vi "RT.vi"() -> ()   [LabVIEW 2013]
uses:
  ieeeC37_118.dll
  pmuConnectionData.dll
  <vilib>/rvi/interface/nirviOpenFPGA/nirviOpenFPGA.xnode
  <vilib>/rvi/interface/nirviReadWriteControl/nirviReadWriteControl.xnode
  <vilib>/rvi/interface/nirviCloseFPGA/nirviCloseFPGA.xnode
  <vilib>/FPGAPlugInAG/Dynamic/niLvFpga_Close_Dynamic.vi
  FPGA Bitfiles/AudurPhasorPodKh_FPGATarget_FPGA_S0BGwwaa7CI.lvbitx
  FPGA.vi
  <vilib>/FPGAPlugInAG/cRIO-9081/niLvFpga_Open_cRIO-9081.vi
  <vilib>/rvi/interface/common/dynamic/niFpgaDynamicAddResources.vi
  NiFpgaLv.dll
  <vilib>/Utility/error.llb/Error Cluster From Error Code.vi
  <vilib>/rvi/interface/Simulation/niFpgaSimulationCallBeginRW.vi
  <vilib>/rvi/errors/niLvFpgaAdjustHostInterfaceError.vi
panel:
  in  "Scaling":sgl
  in  "Alpha":sgl
  in  "Freq of Osc":sgl
  out "FPGA error":errorcluster
  out "Samples\nReceived":i32
  in  "Tab Control 4":enum32{"PMUs Data Stream"}(tab)
  out "Frequency":sgl[](array[numeric])
  out "ROCOF":sgl[](array[numeric])
  out "Phasors\n(Magnitude)":sgl[](array[numeric])
  out "Phasors\n(Angle-Degree)":sgl[](array[numeric])
  out "Data Time Stamp":T1
  out "Analogs\n(Value)":sgl[](array[numeric])
  out "Phasors\n(Channel Names)":string[](array[string])
  out "Phasors\n(Types)":string[](array[string])
  out "Phasors\n(PMU Names)":string[](array[string])
  out "Analogs\n(Channel Names)":string[](array[string])
  out "Analogs\n(Types)":string[](array[string])
  out "Analogs\n(PMU Names)":string[](array[string])
  out "Data Error Status":string[](array[string])
  out "PMU Sync Status":string[](array[string])
  out "Data Processed":string[](array[string])
  out "PMU Time Quality":string[](array[string])
  out "PMU Unlocked Time":string[](array[string])
  out "PMU Triggered":string[](array[string])
  out "Trigger Reason":string[](array[string])
  in  "Tab Control 3":enum32{"Connection Data"}(tab)
  in  "IP Address (PMU / PDC)":string="130.237.53.177"
  in  "ID CODE":i32=787
  in  "Port Number":i32=38068
  in  "Tab Control 2":enum32{"PMUs Configuration"}(tab)
  out "Number of\nAnalogs":u16[](array[numeric])
  out "Number of\nDigitals":u16[](array[numeric])
  out "Nominal\nFrequency":sgl[](array[numeric])
  out "Configuration\nCount":u16[](array[numeric])
  out "Number of\nPhasors":u16[](array[numeric])
  out "Station\nName":string[](array[string])
  out "ID Code":u16[](array[numeric])
  in  "Tab Control":enum32{"PDC Configuration"}(tab)
  out "Data Rate:":u16
  out "Number of PMUs:":u16
  out "Configuration Time Stamp":T2
  in  "Shut Down":bool
  out "error out":errorcluster
  # "FPGA Controlls"
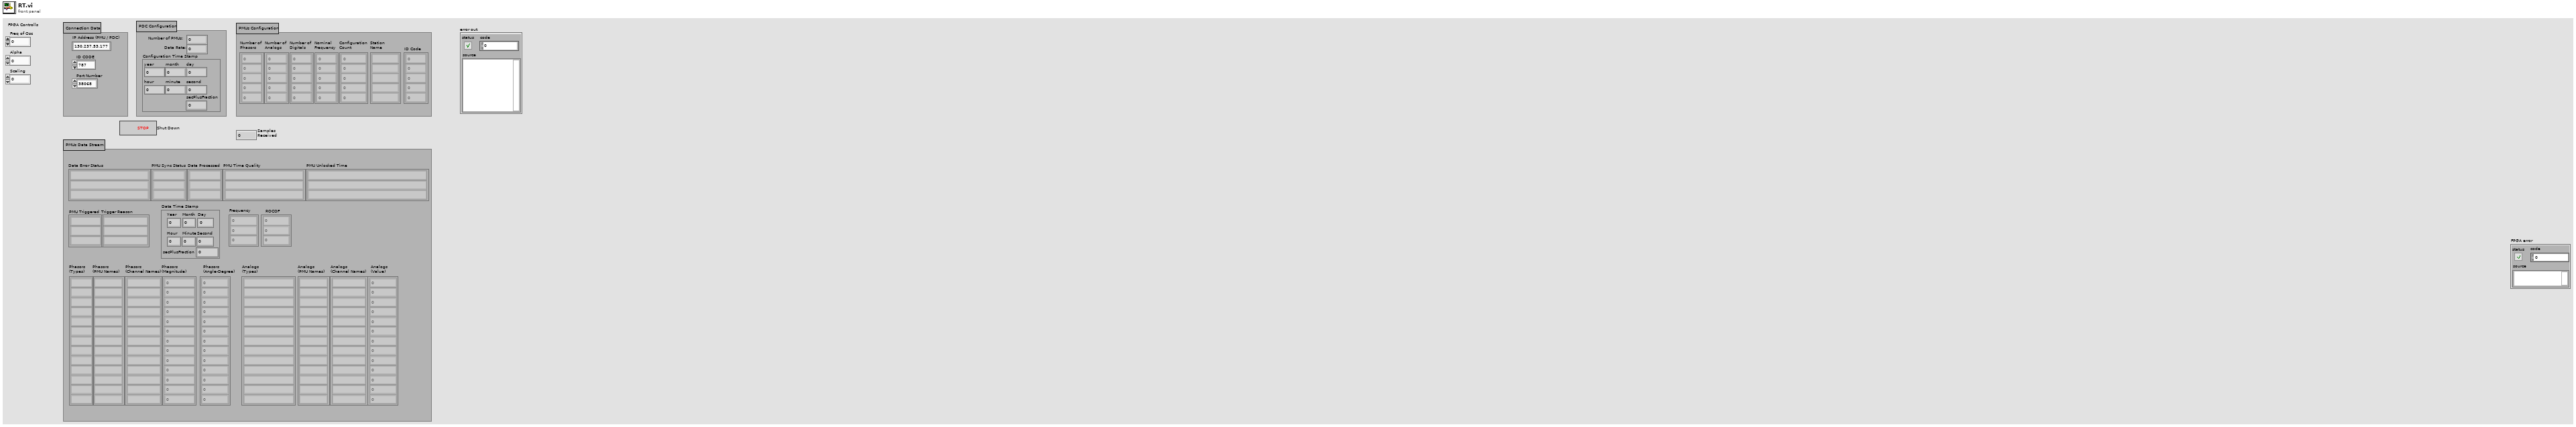
[diagram p1: front panel]
types:
  T1 = cluster{"Year":i32, "Month":i32, "Day":i32, "Hour":i32, "Minute":i32, "Second":i32, "secPlusFraction":sgl}
  T2 = cluster{"year":i32, "month":i32, "day":i32, "hour":i32, "minute":i32, "second":i32, "secPlusFraction":sgl}
  T3 = cluster{"dataError":u8, "dataModified":u8, "pmuIsNOTSync":u8, "pmuIsTriggered":u8, "pmuTimeQuality":u8, "triggerReason":u8, "unlockTime":u8}
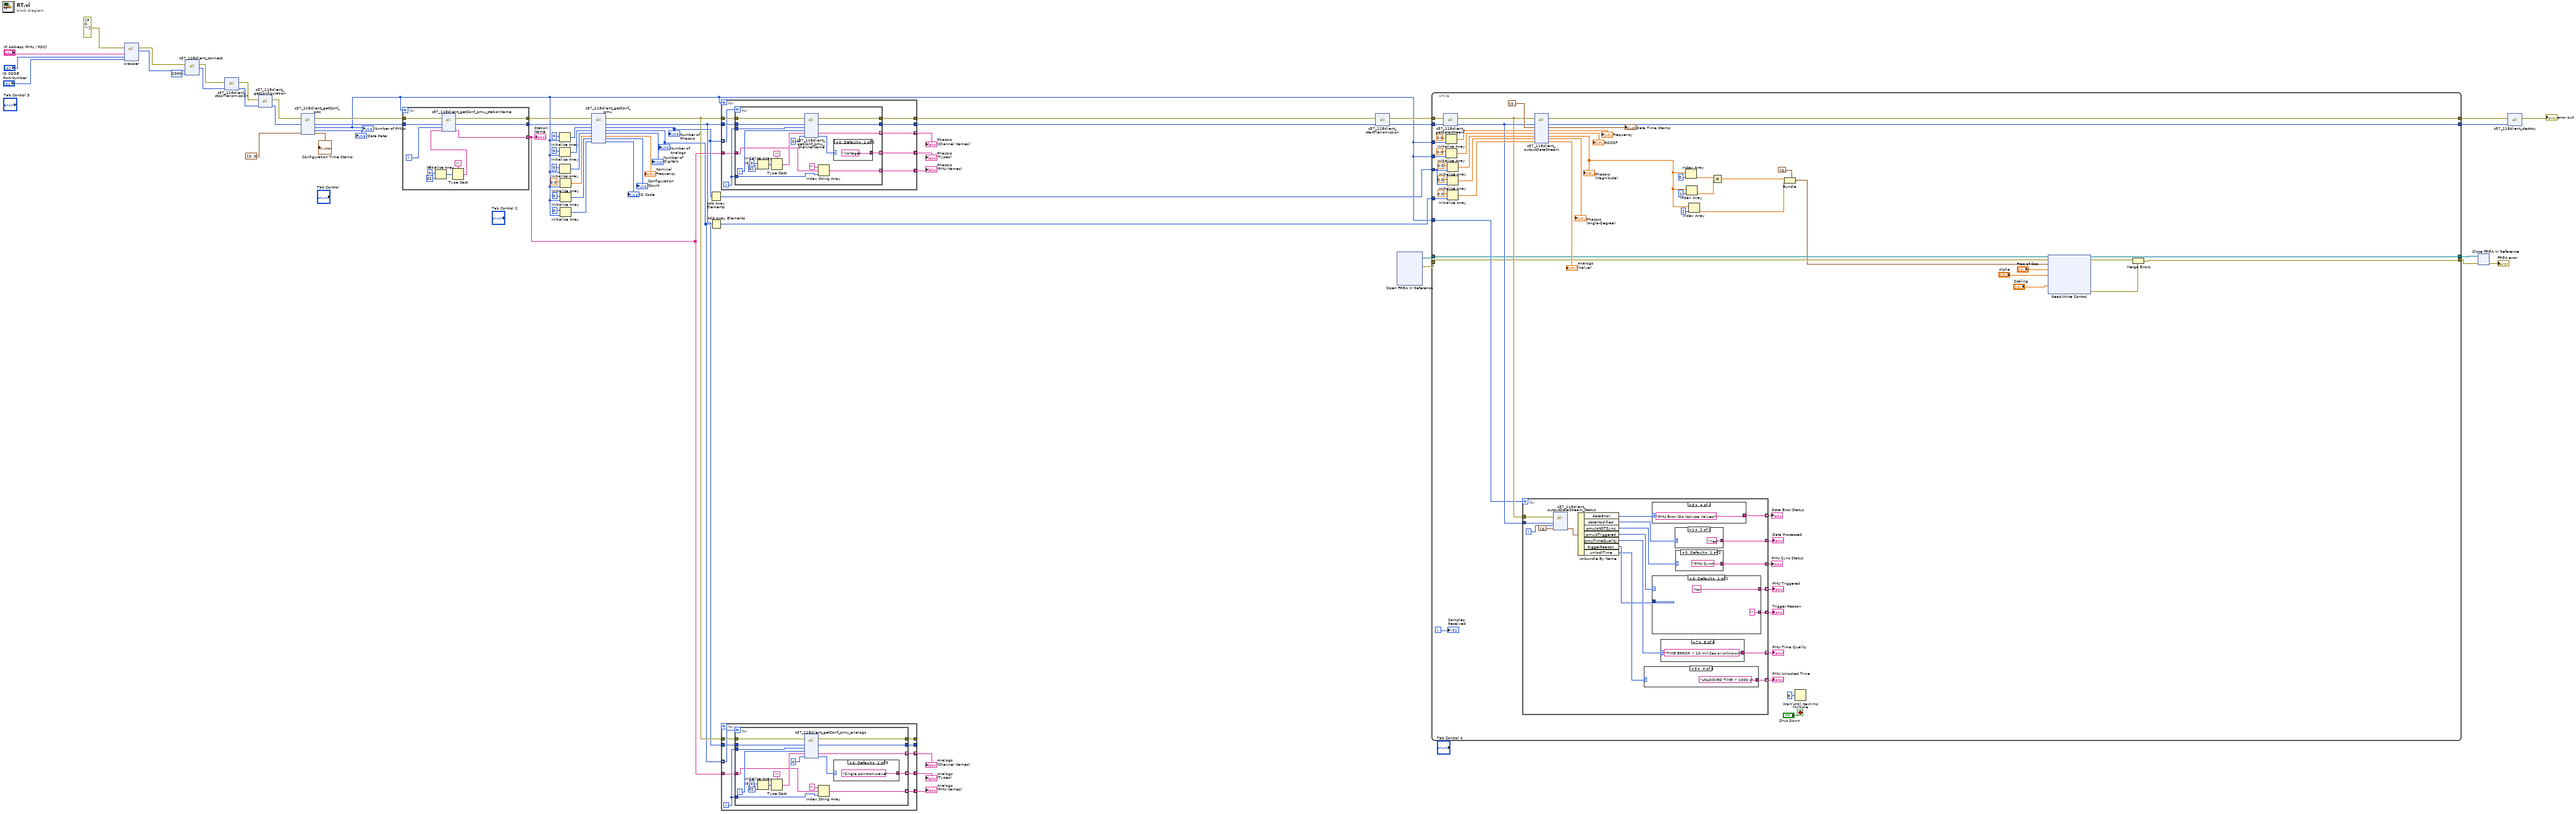
[diagram p0: block diagram]
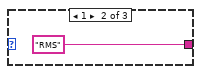
[diagram p2: hidden frame]
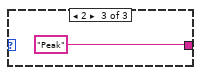
[diagram p3: hidden frame]
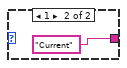
[diagram p4: hidden frame]
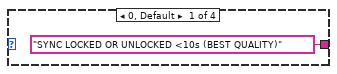
[diagram p5: hidden frame]
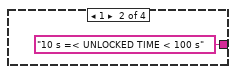
[diagram p6: hidden frame]
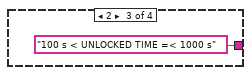
[diagram p7: hidden frame]
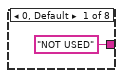
[diagram p8: hidden frame]
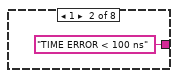
[diagram p9: hidden frame]
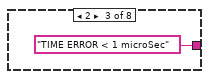
[diagram p10: hidden frame]
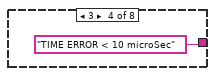
[diagram p11: hidden frame]
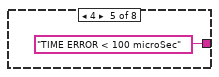
[diagram p12: hidden frame]
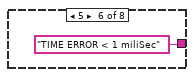
[diagram p13: hidden frame]
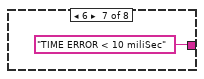
[diagram p14: hidden frame]
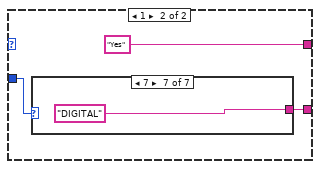
[diagram p15: hidden frame]
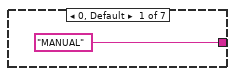
[diagram p16: hidden frame]
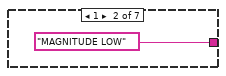
[diagram p17: hidden frame]
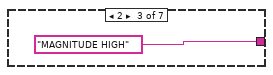
[diagram p18: hidden frame]
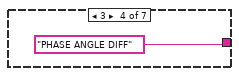
[diagram p19: hidden frame]
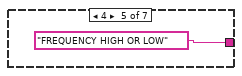
[diagram p20: hidden frame]
diagram:
  n1 = dll-call lib="pmuConnectionData.*" fn="wrapper"(error in=errorcluster {"status"=FALSE, "code"=0, "source"=""} ("error in (no error)"), "ipAddress_PmuServer"="IP Address (PMU / PDC)", "pmuPortNumber"="ID CODE", "pmuIdCode"="Port Number") -> (error out=w53:errorcluster, "PMUConnectionData"=w62:i64)  [unwired: 5 in, 1 out]
  n2 = dll-call lib="ieeeC37_118.*" fn="c37_118client_connect"(error in=w53, "parameters"=w62, "timeoutInMs"=u32 2000) -> (error out=w52:errorcluster, "c37_118Object"=w60:i64)  [unwired: 4 in, 1 out]
  n3 = dll-call lib="ieeeC37_118.dll" fn="c37_118client_stopTransmission"(error in=w52, "self"=w60) -> (error out=w51:errorcluster, "self"=w59:i64)  [unwired: 3 in, 1 out]
  n4 = dll-call lib="ieeeC37_118.dll" fn="c37_118client_getConfiguration"(error in=w51, "self"=w59) -> (error out=w50:errorcluster, "self"=w56:i64)  [unwired: 3 in, 1 out]
  n5 = dll-call lib="ieeeC37_118.dll" fn="c37_118client_getConf_pdc"(error in=w50, "self"=w56, "timestamp"=T2 {"year"=0, "month"=0, "day"=0, "hour"=0, "minute"=0, "second"=0, "secPlusFraction"=0.0}) -> (error out=w27:errorcluster, "self"=w25:i64, "num_pmu"=w6:u16, "data_rate"=→"Data Rate:":u16, "timestamp"=→"Configuration Time Stamp":T2)  [unwired: 5 in, 1 out]
  "Number of PMUs:" <- w6
  n6 = for {
    N: w6 -> [_]
    tunnel: w27 -> [w73]
    tunnel: [w72] -> w26
    tunnel: w25 -> [w71]
    tunnel: [w70] -> w24
    tunnel: [w69] -> w10 mode=indexing
    i -> [w63]
    w68 = i8 0  # I8
    n7 = Initialize Array(w68, 32 ("dimension size")) -> (w67:i8[])
    n8 = Type Cast(type="", x=w67) -> (*(type *) &x=w65:string)
    n9 = dll-call lib="ieeeC37_118.dll" fn="c37_118client_getConf_pmu_stationName"(error in=w73, "self"=w71, "pmuNumber"=w63, "stationName"=w65) -> (error out=w72:errorcluster, "self"=w70:i64, "stationName"=w69:string)  [unwired: 4 in, 1 out]
  }
  "Station\nName" <- w10
  n10 = Initialize Array(u16 0 ("element"), w6) -> (w43:u16[])
  n11 = Initialize Array(u16 0 ("element"), w6) -> (w40:u16[])
  n12 = Initialize Array(u16 0 ("element"), w6) -> (w36:u16[])
  n13 = Initialize Array(sgl 0.0 ("element"), w6) -> (w35:sgl[])
  n14 = Initialize Array(u16 0 ("element"), w6) -> (w34:u16[])
  n15 = Initialize Array(u16 0 ("element"), w6) -> (w17:u16[])
  n16 = dll-call lib="ieeeC37_118.dll" fn="c37_118client_getConf_pmu"(error in=w26, "self"=w24, "numPhasors"=w43, "numAnalog"=w40, "numdigital"=w36, "freqNom"=w35, "configCount"=w34, "idCode"=w17) -> (error out=w9:errorcluster, "self"=w7:i64, "numPhasors"=w21:u16[], "numAnalog"=w8:u16[], "numdigital"=→"Number of\nDigitals":u16[], "freqNom"=→"Nominal\nFrequency":sgl[], "configCount"=→"Configuration\nCount":u16[], "idCode"=→"ID Code":u16[])  [unwired: 3 in, 1 out]
  "Number of\nAnalogs" <- w8
  "Number of\nPhasors" <- w21
  n17 = Add Array Elements(numeric array=w21) -> (sum=w23:u16)
  n18 = Add Array Elements(numeric array=w8) -> (sum=w28:u16)
  n19 = for {
    N: w6 -> [_]
    tunnel: w9 -> [w82]
    tunnel: [w81] -> w11
    tunnel: w7 -> [w83]
    tunnel: [w80] -> w12
    tunnel: [w79] -> w22 mode=concatenating
    tunnel: w21 -> [w78] mode=indexing
    tunnel: [w77] -> w20 mode=concatenating
    tunnel: w10 -> [w76]
    tunnel: [w74] -> w19 mode=concatenating
    i -> [w75]
    n20 = for {
      N: w78 -> [_]
      tunnel: w75 -> [w96]
      tunnel: w83 -> [w95]
      tunnel: w82 -> [w94]
      tunnel: [w93] -> w81
      tunnel: [w92] -> w80
      tunnel: [w91] -> w79 mode=indexing
      tunnel: [w88] -> w77 mode=indexing
      tunnel: w76 -> [w86]
      tunnel: w75 -> [w87]
      tunnel: [w84] -> w74 mode=indexing
      i -> [w97]
      w102 = i8 0  # I8
      n21 = Initialize Array(w102, 32 ("dimension size")) -> (w101:i8[])
      n22 = Type Cast(type="", x=w101) -> (*(type *) &x=w98:string)
      n23 = dll-call lib="ieeeC37_118.dll" fn="c37_118client_getConf_pmu_channelName"(error in=w94, "self"=w95, "pmuNumber"=w96, "phasor"=w97, "channelName"=w98, "phasorType"=0) -> (error out=w93:errorcluster, "self"=w92:i64, "channelName"=w91:string, "phasorType"=w89:i32)  [unwired: 5 in, 1 out]
      n24 = Index String Array(1:w87, 2:w86, 3:"" ("string (\"\")")) -> (0:w84:string)
      n25 = case shown="0, Default" w89 {
        tunnel: ["Voltage" "Current"] -> w88
        frame 0, Default {
        }
        frame 1 {
        }
      }
    }
  }
  "Phasors\n(Channel Names)" <- w22
  "Phasors\n(Types)" <- w20
  "Phasors\n(PMU Names)" <- w19
  n26 = for {
    tunnel: w9 -> [w113]
    tunnel: [w112] -> _
    tunnel: w7 -> [w114]
    tunnel: [w111] -> _
    tunnel: [w110] -> w15 mode=concatenating
    tunnel: w8 -> [w109] mode=indexing
    tunnel: [w108] -> w14 mode=concatenating
    tunnel: w10 -> [w107]
    tunnel: [w105] -> w13 mode=concatenating
    i -> [w106]
    n27 = for {
      N: w109 -> [_]
      tunnel: w106 -> [w127]
      tunnel: w114 -> [w126]
      tunnel: w113 -> [w125]
      tunnel: [w124] -> w112
      tunnel: [w123] -> w111
      tunnel: [w122] -> w110 mode=indexing
      tunnel: [w119] -> w108 mode=indexing
      tunnel: w107 -> [w117]
      tunnel: w106 -> [w118]
      tunnel: [w115] -> w105 mode=indexing
      i -> [w128]
      w133 = i8 0  # I8
      n28 = Initialize Array(w133, 32 ("dimension size")) -> (w132:i8[])
      n29 = Type Cast(type="", x=w132) -> (*(type *) &x=w129:string)
      n30 = dll-call lib="ieeeC37_118.dll" fn="c37_118client_getConf_pmu_analogs"(error in=w125, "self"=w126, "pmuNumber"=w127, "analog"=w128, "channelName"=w129, "analogType"=0 ("phasorType")) -> (error out=w124:errorcluster, "self"=w123:i64, "channelName"=w122:string, "analogType"=w120:i32)  [unwired: 5 in, 1 out]
      n31 = Index String Array(1:w118, 2:w117, 3:"" ("string (\"\")")) -> (0:w115:string)
      n32 = case shown="0, Default" w120 {
        tunnel: ["Single point-on-wave" "RMS" "Peak"] -> w119
        frame 0, Default {
        }
        frame 1 {
        }
        frame 2 {
        }
      }
    }
  }
  "Analogs\n(Channel Names)" <- w15
  "Analogs\n(Types)" <- w14
  "Analogs\n(PMU Names)" <- w13
  n33 = dll-call lib="ieeeC37_118.dll" fn="c37_118client_startTransmission"(error in=w11, "self"=w12) -> (error out=w49:errorcluster, "self"=w58:i64)  [unwired: 3 in, 1 out]
  n34 = xnode "Open FPGA VI Reference"() -> ("FPGA VI Reference Out"=w5:refnum<k20>, "error out"=w4:errorcluster)  [unwired: 2 in]
  n35 = while {
    tunnel: w58 -> [w192]
    tunnel: [w187] -> w57
    tunnel: w49 -> [w190]
    tunnel: [w189] -> w48
    tunnel: w6 -> [w185]
    tunnel: w6 -> [w182]
    tunnel: w23 -> [w176]
    tunnel: w28 -> [w169]
    tunnel: w6 -> [w165]
    tunnel: w5 -> [w149]
    tunnel: w4 -> [w148]
    tunnel: [w147] -> w2
    tunnel: [w137] -> w1
    i -> [w171]
    stop <- "Shut Down" stop-if-true
    n36 = dll-call lib="ieeeC37_118.dll" fn="c37_118client_getDataStream"(error in=w190, "self"=w192) -> (error out=w166:errorcluster, "self"=w167:i64)  [unwired: 3 in, 1 out]
    n37 = Initialize Array(sgl 0.0 ("element"), w185) -> (w184:sgl[])
    n38 = Initialize Array(sgl 0.0 ("element"), w182) -> (w181:sgl[])
    n39 = Initialize Array(sgl 0.0 ("element"), w176) -> (w175:sgl[])
    n40 = Initialize Array(sgl 0.0 ("element"), w176) -> (w174:sgl[])
    n41 = Initialize Array(sgl 0.0 ("element"), w169) -> (w168:sgl[])
    n42 = for {
      N: w165 -> [_]
      tunnel: w167 -> [w211]
      tunnel: w166 -> [w210]
      tunnel: [w207] -> w164 mode=indexing
      tunnel: [w204] -> w163 mode=indexing
      tunnel: [w201] -> w162 mode=indexing
      tunnel: [w199] -> w161 mode=indexing
      tunnel: [w198] -> w160 mode=indexing
      tunnel: [w195] -> w159 mode=indexing
      tunnel: [w193] -> w158 mode=indexing
      i -> [w209]
      n43 = dll-call lib="ieeeC37_118.dll" fn="c37_118client_outputDataStream_status"(error in=w210, "self"=w211, "pmuNumber"=w209, "status"=T3 {"dataError"=0, "dataModified"=0, "pmuIsNOTSync"=0, "pmuIsTriggered"=0, "pmuTimeQuality"=0, "triggerReason"=0, "unlockTime"=0}) -> ("status"=w206:T3)  [unwired: 5 in, 2 out]
      n44 = Unbundle By Name(w206) -> ("dataError"=w203:u8, "dataModified"=w202:u8, "pmuIsNOTSync"=w205:u8, "pmuIsTriggered"=w200:u8, "pmuTimeQuality"=w197:u8, "triggerReason"=w196:u8, "unlockTime"=w194:u8)
      n45 = case shown="3" w194 {
        tunnel: ["SYNC LOCKED OR UNLOCKED <10s (BEST QUALITY)" "10 s =< UNLOCKED TIME < 100 s" "100 s < UNLOCKED TIME =< 1000 s" "UNLOCKED TIME > 1000 s"] -> w193
        frame 0, Default {
        }
        frame 1 {
        }
        frame 2 {
        }
        frame 3 {
        }
      }
      n46 = case shown="3" w203 {
        tunnel: ["Good Measurment Data (No Errors)" "PMU Error, No Information About Data" "PMU In Test Mode (Do Not Use Values)" "PMU Error (Do Not Use Values)"] -> w207
        frame 0, Default {
        }
        frame 1 {
        }
        frame 2 {
        }
        frame 3 {
        }
      }
      n47 = case shown="0, Default" w200 {
        tunnel: ["No" "Yes"] -> w199
        tunnel: w196 -> [_ w227]
        tunnel: ["" w226] -> w195
        frame 0, Default {
        }
        frame 1 {
          n48 = case shown="7" w227 {
            tunnel: ["MANUAL" "MAGNITUDE LOW" "MAGNITUDE HIGH" "PHASE ANGLE DIFF" "FREQUENCY HIGH OR LOW" "df/dt HIGH" "DIGITAL"] -> w226
            frame 0, Default {
            }
            frame 1 {
            }
            frame 2 {
            }
            frame 3 {
            }
            frame 4 {
            }
            frame 5 {
            }
            frame 7 {
            }
          }
        }
      }
      n49 = case shown="7" w197 {
        tunnel: ["NOT USED" "TIME ERROR < 100 ns" "TIME ERROR < 1 microSec" "TIME ERROR < 10 microSec" "TIME ERROR < 100 microSec" "TIME ERROR < 1 miliSec" "TIME ERROR < 10 miliSec" "TIME ERROR > 10 miliSec or Unknown"] -> w198
        frame 0, Default {
        }
        frame 1 {
        }
        frame 2 {
        }
        frame 3 {
        }
        frame 4 {
        }
        frame 5 {
        }
        frame 6 {
        }
        frame 7 {
        }
      }
      n50 = case shown="1" w202 {
        tunnel: ["No" "Yes"] -> w201
        frame 0, Default {
        }
        frame 1 {
        }
      }
      n51 = case shown="0, Default" w205 {
        tunnel: ["PMU Sync" "PMU Not Sync"] -> w204
        frame 0, Default {
        }
        frame 1 {
        }
      }
    }
    "Data Error Status" <- w164
    "PMU Sync Status" <- w163
    "Data Processed" <- w162
    "PMU Triggered" <- w161
    "PMU Time Quality" <- w160
    "Trigger Reason" <- w159
    "PMU Unlocked Time" <- w158
    n52 = dll-call lib="ieeeC37_118.dll" fn="c37_118client_outputDataStream"(error in=w166, "self"=w167, "timestamp"=T2 {"year"=0, "month"=0, "day"=0, "hour"=0, "minute"=0, "second"=0, "secPlusFraction"=0.0}, "freqBuffer"=w184, "rocofBuffer"=w181, "phasorsMagBuffer"=w175, "phasorsAngBuffer"=w174, "analogBuffer"=w168) -> (error out=w189:errorcluster, "self"=w187:i64, "timestamp"=→"Data Time Stamp":T2, "freqBuffer"=→"Frequency":sgl[], "rocofBuffer"=→"ROCOF":sgl[], "phasorsMagBuffer"=w146:sgl[], "phasorsAngBuffer"=→"Phasors\n(Angle-Degree)":sgl[], "analogBuffer"=→"Analogs\n(Value)":sgl[])  [unwired: 3 in, 1 out]
    "Phasors\n(Magnitude)" <- w146
    n53 = Index Array(array=w146, index=0) -> (element=w153:sgl)
    n54 = Index Array(array=w146, index=1) -> (element=w152:sgl)
    n55 = Index Array(array=w146, index=2) -> (element=w145:sgl)
    n56 = Multiply(x=w153, y=w152) -> (x*y=w150:sgl)
    n57 = Bundle(cluster=cluster{sgl, sgl} {0.0, 0.0}, w150, w145) -> (w143:cluster{sgl, sgl})
    n58 = Wait Until Next ms Multiple(millisecond multiple=u32 5) -> ()  [unwired: 1 out]
    n59 = xnode "Read/Write Control"("FPGA VI Reference In"=w149, "error in"=w148, "PMU measurments"=w143, "Freq of Osc"="Freq of Osc", "Alpha"="Alpha", "Scaling"="Scaling") -> ("FPGA VI Reference Out"=w147:refnum<k20>, "error out"=w139:errorcluster, "FPGA Error Out"=w138:errorcluster)  [unwired: 1 in]
    n60 = Merge Errors(w139, w138) -> (w137:errorcluster)
    "Samples\nReceived" <- w171
  }
  n61 = xnode "Close FPGA VI Reference"("FPGA VI Reference In"=w2, "error in"=w1) -> ("error out"=→"FPGA error":errorcluster)
  n62 = dll-call lib="ieeeC37_118.dll" fn="c37_118client_destroy"(error in=w48, "self"=w57) -> (error out=→"error out":errorcluster)  [unwired: 4 in, 1 out]
